vi "Kinect_Raw_Depth_to_Meters_Double.vi"(4 "Raw":dbl) -> (1 "Meters":dbl)   [LabVIEW 2011]
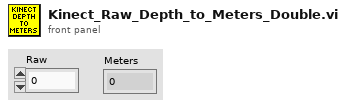
[diagram p1: front panel]
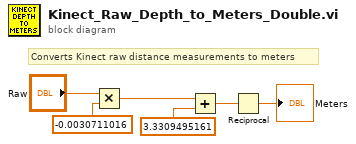
[diagram p0: block diagram]
diagram:
  # "Converts Kinect raw distance measurements to meters"
  n1 = Multiply(x="Raw", y=-0.0030711016) -> (x*y=w5:dbl)
  n2 = Add(x=w5, y=3.3309495161) -> (x+y=w3:dbl)
  n3 = Reciprocal(x=w3) -> (1/x=→"Meters":dbl)
